vi "access angular position.vi"(9 "Z angle":dbl, 10 "Y angle":dbl, 11 "x angle":dbl) -> (2 "Value":T1 items=["XY Plane", "XZ Plane", "YZ Plane", "arbitraryplane"], 3 "Angle":dbl)   [LabVIEW 2020]
uses:
  Typedefs/Plane Mode.ctl
panel:
  out "number":u32
  out "appended array":bool[](array[boolean])
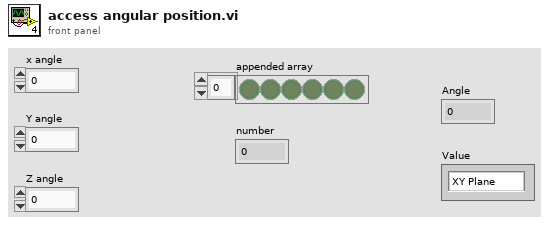
[diagram p1: front panel]
types:
  T1 = typedef "Plane Mode.ctl" = u16
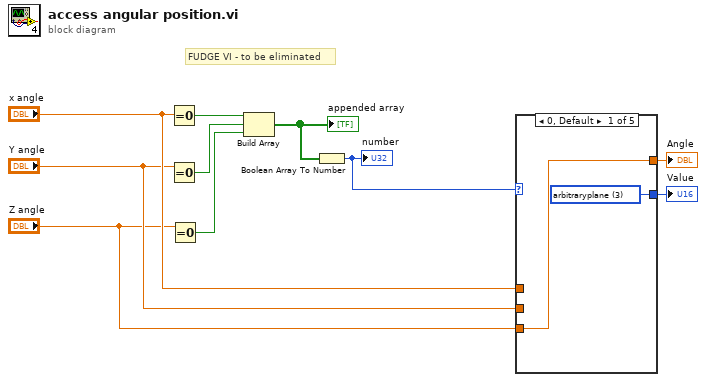
[diagram p0: block diagram]
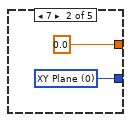
[diagram p2: hidden frame]
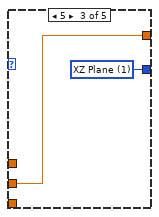
[diagram p3: hidden frame]
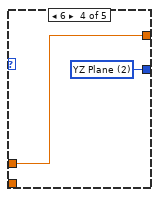
[diagram p4: hidden frame]
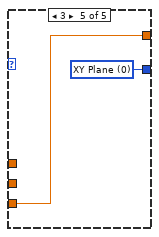
[diagram p5: hidden frame]
diagram:
  # "FUDGE VI - to be eliminated"
  n1 = Equal To 0?(x="x angle") -> (x = 0?=w10:bool)
  n2 = Equal To 0?(x="Y angle") -> (x = 0?=w9:bool)
  n3 = Equal To 0?(x="Z angle") -> (x = 0?=w8:bool)
  n4 = Build Array(w10, w9, w8) -> (w7:bool[])
  "appended array" <- w7
  n5 = Boolean Array To Number(Boolean array=w7) -> (number=w6:u32)
  "number" <- w6
  n6 = case shown="0, Default" w6 {
    tunnel: [w12 0.0 w16 w18 w20] -> w4
    tunnel: [w11 w13 w15 w17 w19] -> w5
    tunnel: "x angle" -> [_ _ _ w18 _]
    tunnel: "Y angle" -> [_ _ w16 _ _]
    tunnel: "Z angle" -> [w12 _ _ _ w20]
    frame 0, Default {
      w11 = T1 3 items=["XY Plane", "XZ Plane", "YZ Plane", "arbitraryplane"] ("Value")
    }
    frame 7 {
      w13 = T1 0 items=["XY Plane", "XZ Plane", "YZ Plane", "arbitraryplane"] ("Value")
    }
    frame 5 {
      w15 = T1 1 items=["XY Plane", "XZ Plane", "YZ Plane", "arbitraryplane"] ("Value")
    }
    frame 6 {
      w17 = T1 2 items=["XY Plane", "XZ Plane", "YZ Plane", "arbitraryplane"] ("Value")
    }
    frame 3 {
      w19 = T1 0 items=["XY Plane", "XZ Plane", "YZ Plane", "arbitraryplane"] ("Value")
    }
  }
  "Value" <- w5
  "Angle" <- w4
